vi "AddCredit.vi"(8 "error in (no error)":errorcluster, 10 "Credit Added":dbl, 11 "UI Actor in":refnum<class "UI Actor.lvclass">) -> (0 "error out":errorcluster, 3 "UI Actor out":refnum<class "UI Actor.lvclass">)   [LabVIEW 2020, in "UI Actor.lvlib" / "UI Actor.lvclass"]
uses:
  UI Actor.lvclass
  UI Actor.lvclass/UI Actor.ctl
  Messages Actor Messages/AddCredit Msg/AddCredit Msg.lvclass/AddCredit Msg.ctl
  <vilib>/ActorFramework/Message Enqueuer/Message Enqueuer.lvclass/Message Enqueuer.ctl
  <vilib>/ActorFramework/Message Enqueuer/Enqueue.vi
  Messages Actor Messages/AddCredit Msg/AddCredit Msg.lvclass
  C:/Program Files (x86)/National Instruments/LabVIEW 2020/vi.lib/ActorFramework/Message/Message.lvclass
  <vilib>/ActorFramework/Message Priority Queue/Priority Enqueue.vi
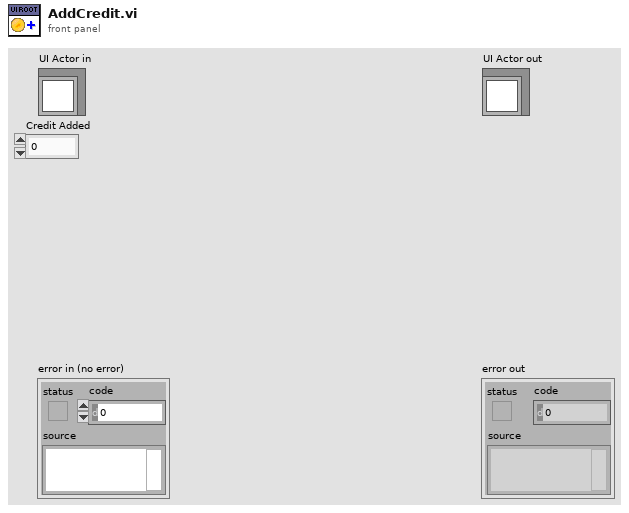
[diagram p1: front panel]
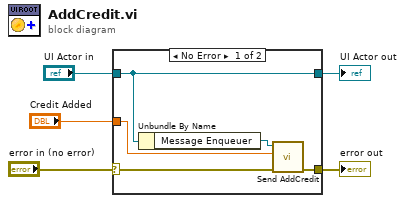
[diagram p0: block diagram]
diagram:
  n1 = case shown="No Error" "error in (no error)" {
    selector: "error in (no error)" -> [w8 w12]
    tunnel: [w7 w12] -> w4
    tunnel: [w10 w11] -> w2
    tunnel: "UI Actor in" -> [w10 w11]
    tunnel: "Credit Added" -> [w6 _]
    frame No Error {
      n2 = Unbundle By Name(w10) -> ("Message Enqueuer"=w9:refnum<class "Message Enqueuer.lvclass">)
      n3 = call "Send AddCredit.vi"("error in (no error)"=w8, "Credit Added"=w6, "Message Enqueuer"=w9) -> ("error out"=w7:errorcluster)  [unwired: 7 in, 1 out]
    }
    frame Error {
    }
  }
  "error out" <- w4
  "UI Actor out" <- w2
